vi "Car Wash.vi"() -> ()   [LabVIEW 2019]
uses:
  Controls/Car Wash Indicators.ctl
  Controls/Wash Options.ctl
  Controls/MachineStates.ctl
  Controls/TimerModes.ctl
panel:
  out "Error Out":errorcluster
  in  "Error In":errorcluster
  in  "Start":bool
  out "Elapsed Time":dbl format="%0.2f"
  in  "stop":bool
  out "Wash Entry":bool
  in  "Wash Options":T1
  in  "Car Position Slider":u8(slide) max=3 scale=0.0..4.0
  out "Car Wash Indicators":T2
  # "Entry Console"
  # "Car Wash Display"
  # "Car Position Simulation"
  # "Pre-Soak\nH-P Wash\nL-P Wax\nSpot Free Rinse"
  # "Underbody Wash\nBug Remover"
  # "Tire Shine\nAir Dry"
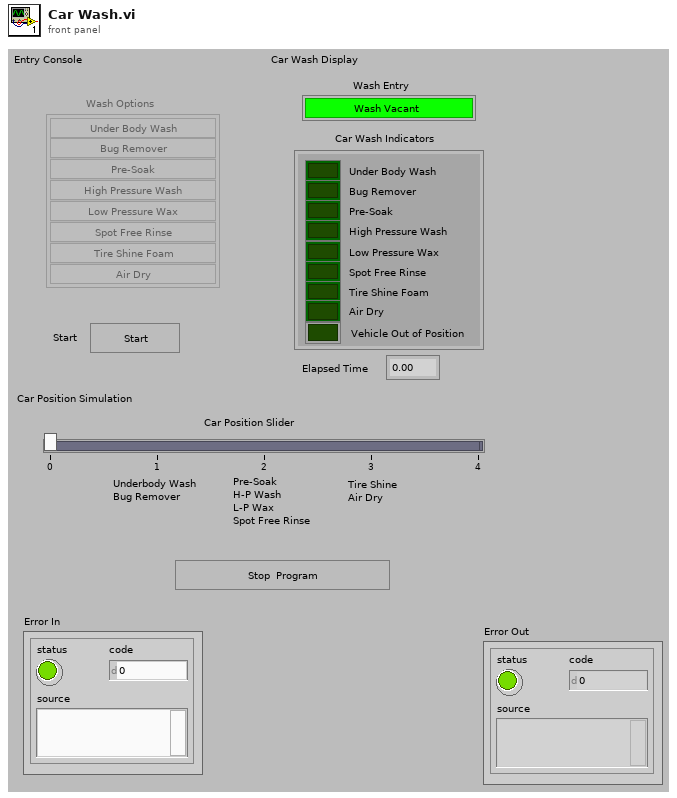
[diagram p1: front panel]
types:
  T1 = typedef "Wash Options.ctl" = cluster{"Underbody Wash":bool, "Bug Remover":bool, "Pre-Soak":bool, "High Pressure Wash":bool, "Low Pressure Wax":bool, "Spot Free Rinse":bool, "Tire Shine Foam":bool, "Air Dry":bool}
  T2 = typedef "Car Wash Indicators.ctl" = cluster{"Under Body Wash":bool, "Bug Remover":bool, "Pre-Soak":bool, "High Pressure Wash":bool, "Low Pressure Wax":bool, "Spot Free Rinse":bool, "Tire Shine Foam":bool, "Air Dry":bool, "Vehicle Out of Position":bool}
  T3 = typedef "MachineStates.ctl" = enum16{"Init", "IDLE", "Start", "Check", "Next", "Pause", "Resume"}
  T4 = enum8{"Enabled", "Disabled", "Disabled and Grayed Out"}
  T5 = typedef "TimerModes.ctl" = enum16{"Start Timer", "Read Time", "Pause", "Resume"}
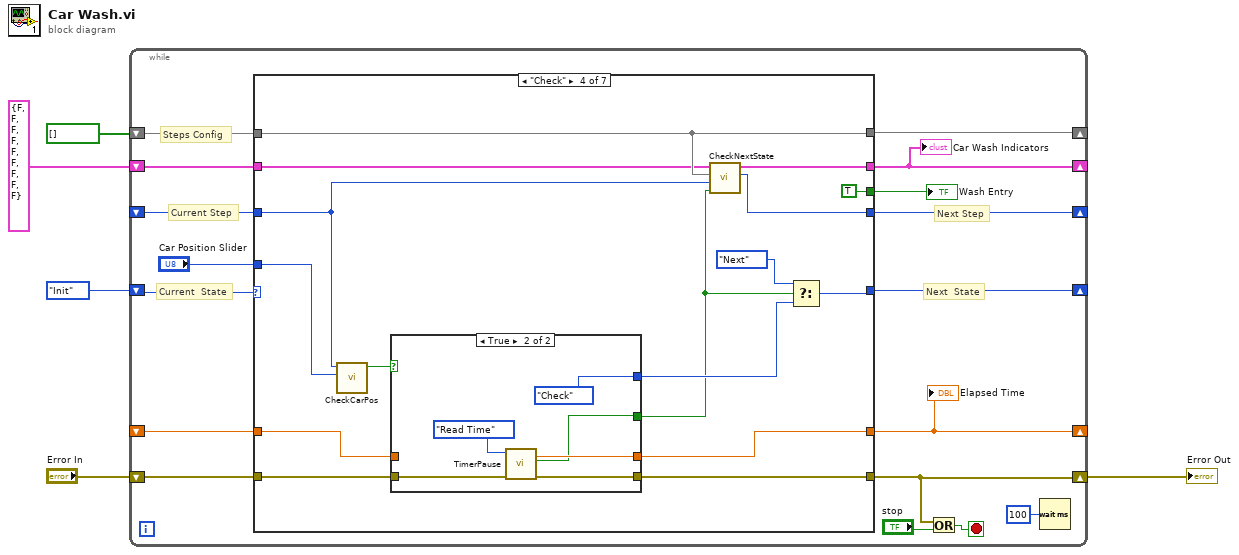
[diagram p0: block diagram]
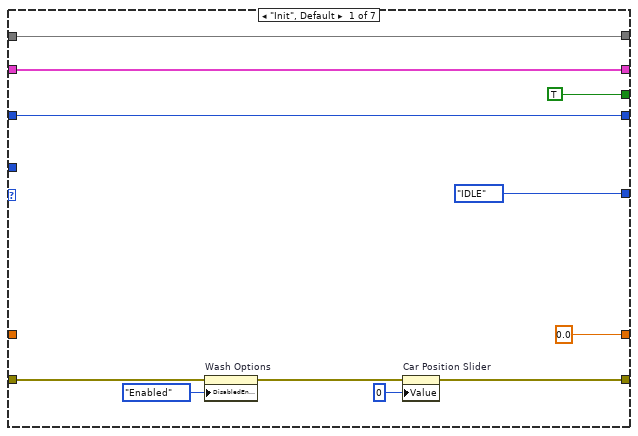
[diagram p2: hidden frame]
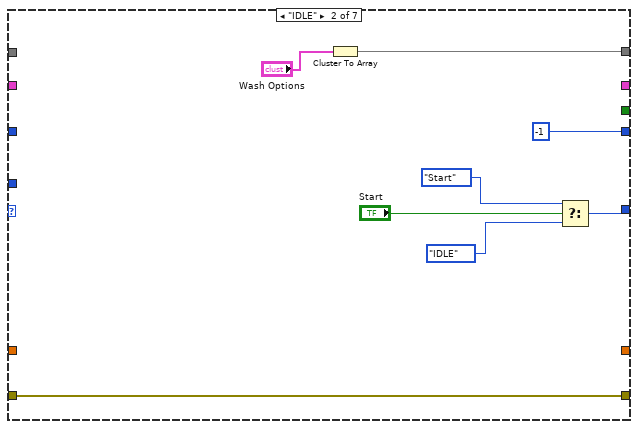
[diagram p3: hidden frame]
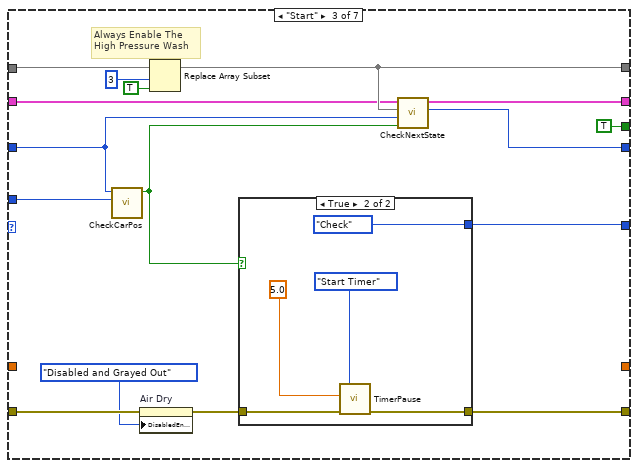
[diagram p4: hidden frame]
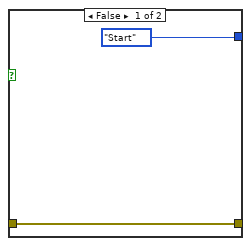
[diagram p5: hidden frame]
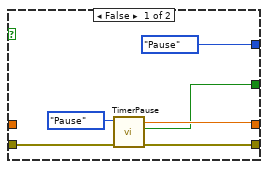
[diagram p6: hidden frame]
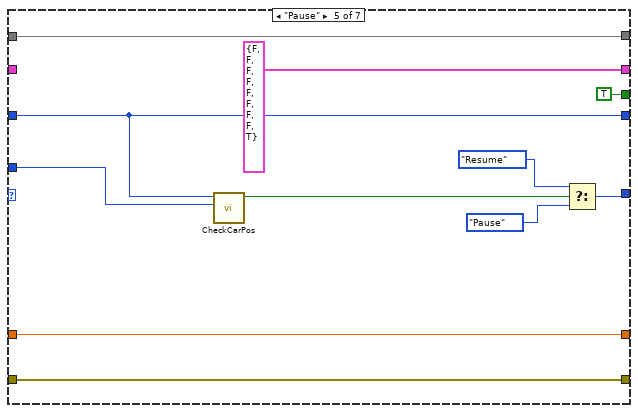
[diagram p7: hidden frame]
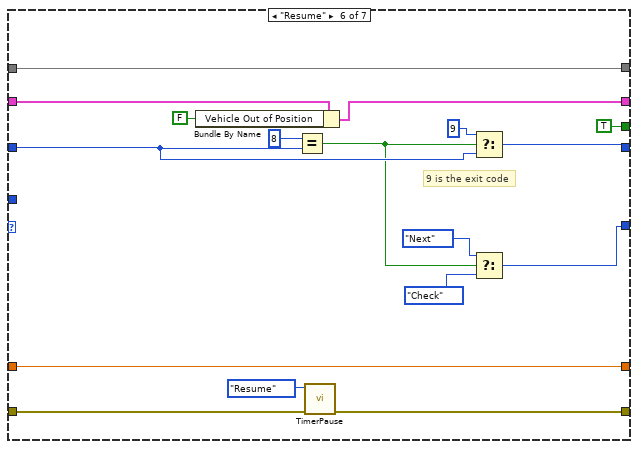
[diagram p8: hidden frame]
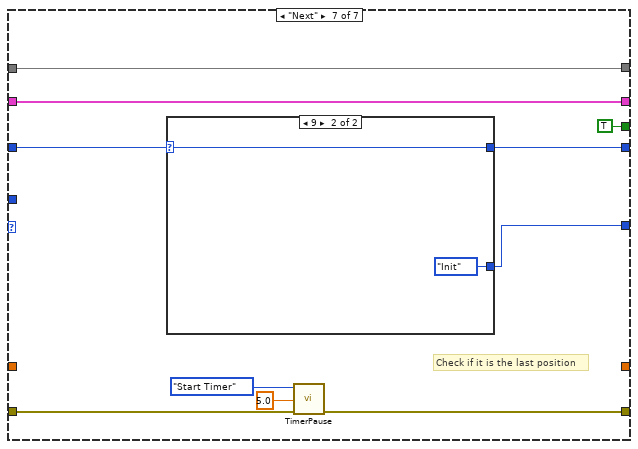
[diagram p9: hidden frame]
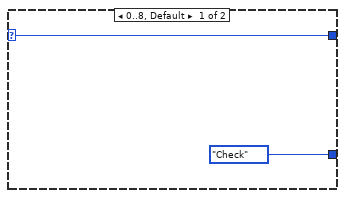
[diagram p10: hidden frame]
diagram:
  n1 = while {
    shift-right: [w17] -> _
    shift-left: MachineStates."Init" -> [w15]
    shift-right: [w9] -> _
    shift-left: bool[] [] ("Wash Options") -> [w16]
    shift-right: [w12] -> _
    shift-left: T2 {"Under Body Wash"=FALSE, "Bug Remover"=FALSE, "Pre-Soak"=FALSE, "High Pressure Wash"=FALSE, "Low Pressure Wax"=FALSE, "Spot Free Rinse"=FALSE, "Tire Shine Foam"=FALSE, "Air Dry"=FALSE, "Vehicle Out of Position"=FALSE} ("Car Wash Indicators") -> [w13]
    shift-right: [w11] -> _
    shift-left: _ -> [w10]
    shift-right: [w8] -> _
    shift-left: _ -> [w7]
    shift-right: [w19] -> w4
    shift-left: "Error In" -> [w20]
    stop <- w22 stop-if-true
    # "Next  State"
    # "Next Step"
    # "Current Step"
    # "Steps Config"
    # "Current  State"
    n2 = case shown="\"Check\"" w15 {
      tunnel: [w26 w41 w54 w78 w95 w117 w126] -> w19
      tunnel: w20 -> [w25 w41 w43 w79 w95 w118 w127]
      tunnel: [0.0 ("Elapsed Time") _ _ w74 w96 w112 _] -> w11
      tunnel: [TRUE ("Wash Entry") _ TRUE ("Wash Entry") TRUE ("Wash Entry") TRUE ("Wash Entry") TRUE ("Wash Entry") TRUE ("Wash Entry")] -> w18
      tunnel: [MachineStates."IDLE" w40 w53 w68 w99 w104 w121] -> w17
      tunnel: w16 -> [w30 _ w52 w75 w103 w120 w130]
      tunnel: [w30 w35 w51 w75 w103 w120 w130] -> w9
      tunnel: "Car Position Slider" -> [_ _ w55 w80 w101 _ _]
      tunnel: w13 -> [w28 _ w50 w73 _ w116 w129]
      tunnel: [w28 _ w49 w72 T2 {"Under Body Wash"=FALSE, "Bug Remover"=FALSE, "Pre-Soak"=FALSE, "High Pressure Wash"=FALSE, "Low Pressure Wax"=FALSE, "Spot Free Rinse"=FALSE, "Tire Shine Foam"=FALSE, "Air Dry"=FALSE, "Vehicle Out of Position"=TRUE} ("Car Wash Indicators") w114 w129] -> w12
      tunnel: w10 -> [_ _ _ w76 w96 w112 _]
      tunnel: [w29 i8 -1 ("Next Position") w48 w71 w94 w111 w122] -> w8
      tunnel: w7 -> [w29 _ w47 w69 w94 w108 w123]
      frame "Init", Default {
        n3 = property on="Wash Options" class="Clust (strict)"(error in=w25, "DisabledEnum"=T4."Enabled" ("Disabled")) -> (error out=w24:errorcluster)  [unwired: 1 in, 1 out]
        n4 = property on="Car Position Slider" class="Slide (strict)"(error in=w24, "Value"=u8 0) -> (error out=w26:errorcluster)  [unwired: 1 in, 1 out]
      }
      frame "IDLE" {
        n5 = Cluster To Array(cluster="Wash Options") -> (array=w35:bool[])
        n6 = Select(t=MachineStates."Start", s="Start", f=MachineStates."IDLE") -> (s? t:f=w40:T3)
      }
      frame "Start" {
        # "Always Enable The \nHigh Pressure Wash"
        n7 = call "CheckCarPos.vi"("Car Position"=w55, "Current Step"=w47) -> ("Position Ok?"=w46:bool)  [unwired: 7 in]
        n8 = property on="Air Dry" class="Bool (strict)"(error in=w43, "DisabledEnum"=T4."Disabled and Grayed Out" ("Disabled")) -> (error out=w44:errorcluster)  [unwired: 1 in, 1 out]
        n9 = Replace Array Subset(array=w52, new element=TRUE ("new element/subarray"), index=3) -> (w51:bool[])
        n10 = case shown="True" w46 {
          tunnel: w44 -> [w59 w62]
          tunnel: [w59 w61] -> w54
          tunnel: [MachineStates."Start" MachineStates."Check"] -> w53
          frame False {
          }
          frame True {
            n11 = call "TimerPause.vi"("Error In"=w62, "Time Target (s)"=5.0, "Timer Mode"=TimerModes."Start Timer") -> ("Error Out"=w61:errorcluster)  [unwired: 6 in, 2 out]
          }
        }
        n12 = call "CheckNextState.vi"("Car Wash IN"=w50, "Wash Options"=w51, "Current Step"=w47, "TimeHasElapsed?"=w46) -> ("Car Wash OUT"=w49:T2, "Next Step"=w48:i8)  [unwired: 5 in]
      }
      frame "Check" {
        n13 = call "CheckCarPos.vi"("Car Position"=w80, "Current Step"=w69) -> ("Position Ok?"=w77:bool)  [unwired: 7 in]
        n14 = case shown="True" w77 {
          tunnel: [w82 w91] -> w74
          tunnel: [w84 w90] -> w78
          tunnel: w79 -> [w85 w89]
          tunnel: [MachineStates."Pause" MachineStates."Check"] -> w66
          tunnel: w76 -> [_ _]
          tunnel: [w81 w87] -> w65
          frame False {
            n15 = call "TimerPause.vi"("Error In"=w85, "Timer Mode"=TimerModes."Pause") -> ("Error Out"=w84:errorcluster, "Has Time Elapsed"=w81:bool, "Elapsed Time (s.ss)"=w82:dbl)  [unwired: 7 in]
          }
          frame True {
            n16 = call "TimerPause.vi"("Error In"=w89, "Timer Mode"=TimerModes."Read Time") -> ("Error Out"=w90:errorcluster, "Has Time Elapsed"=w87:bool, "Elapsed Time (s.ss)"=w91:dbl)  [unwired: 7 in]
          }
        }
        n17 = call "CheckNextState.vi"("Car Wash IN"=w73, "Wash Options"=w75, "Current Step"=w69, "TimeHasElapsed?"=w65) -> ("Car Wash OUT"=w72:T2, "Next Step"=w71:i8)  [unwired: 5 in]
        n18 = Select(t=MachineStates."Next", s=w65, f=w66) -> (s? t:f=w68:T3)
      }
      frame "Pause" {
        n19 = call "CheckCarPos.vi"("Car Position"=w101, "Current Step"=w94) -> ("Position Ok?"=w100:bool)  [unwired: 7 in]
        n20 = Select(t=MachineStates."Resume", s=w100, f=MachineStates."Pause") -> (s? t:f=w99:T3)
      }
      frame "Resume" {
        # "9 is the exit code"
        n21 = Bundle By Name(cluster=w116, "Vehicle Out of Position"=FALSE) -> (w114:T2)
        n22 = Equal?(x=i8 8 ("y"), y=w108) -> (x = y?=w107:bool)
        n23 = call "TimerPause.vi"("Error In"=w118, "Timer Mode"=TimerModes."Resume") -> ("Error Out"=w117:errorcluster)  [unwired: 7 in, 2 out]
        n24 = Select(t=i8 9 ("y"), s=w107, f=w108) -> (s? t:f=w111:i8)
        n25 = Select(t=MachineStates."Next", s=w107, f=MachineStates."Check") -> (s? t:f=w104:T3)
      }
      frame "Next" {
        # "Check if it is the last position"
        n26 = case shown="9" w123 {
          selector: w123 -> [w131 w134]
          tunnel: [MachineStates."Check" MachineStates."Init"] -> w121
          tunnel: [w131 w134] -> w122
          frame 0..8, Default {
          }
          frame 9 {
          }
        }
        n27 = call "TimerPause.vi"("Error In"=w127, "Time Target (s)"=5.0, "Timer Mode"=TimerModes."Start Timer") -> ("Error Out"=w126:errorcluster)  [unwired: 6 in, 2 out]
      }
    }
    "Car Wash Indicators" <- w12
    "Wash Entry" <- w18
    "Elapsed Time" <- w11
    n28 = Or(x=w19, y="stop") -> (x .or. y?=w22:bool)
    n29 = Wait (ms)(milliseconds to wait=u32 100) -> ()  [unwired: 1 out]
  }
  "Error Out" <- w4
